vi "Max-SP-GetChannelRefs.vi"(8 "Error In":errorcluster, 9 "Enabled?":bool, 11 "Device Ref in":T1 format="%.0x") -> (0 "Error Out":errorcluster, 2 "Group Data Array":T2(array[cluster]) {"VS Refs" format="%.0x"}, 3 "Device Ref out":T1=18446744073709551615 format="%.0x")   [LabVIEW 2017, in "Waveform-Processing-Custom-Device Shared.lvlib" / "Max_SP.lvlib"]
uses:
  Max_SP.lvlib
  <vilib>/NI Veristand/Custom Device API/Custom Device Item Ref.ctl
  Constants.vi
  <vilib>/NI Veristand/Custom Device API/Get Item Property (Dependent Node Pointer).vi
  <vilib>/NI Veristand/Custom Device API/Custom Device API.lvlib
  System Explorer/Waveform-Processing-Custom-Device System Explorer.lvlib
  Waveform-Processing-Custom-Device Shared.lvlib
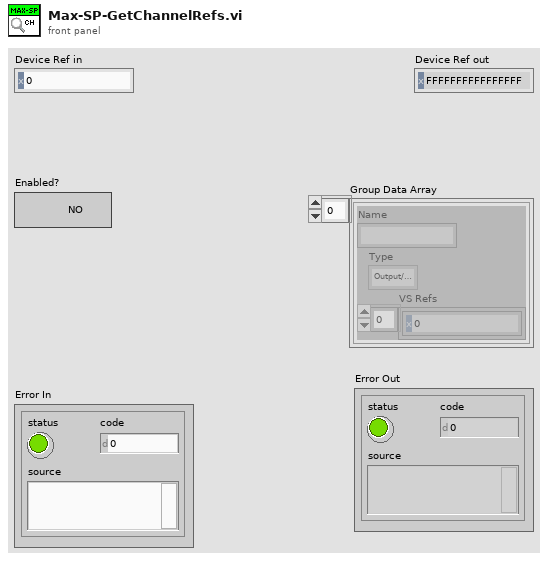
[diagram p1: front panel]
types:
  T1 = typedef "Custom Device API.lvlib/Custom Device Item Ref.ctl" = u64
  T2 = cluster{"Name":string, "Type":enum16{"Output/Write", "Input/Read", "Input/ReadWrite"}, "VS Refs":T1[]}[]
  T3 = enum16{"Output/Write", "Input/Read", "Input/ReadWrite"}
  T4 = cluster{"Name":string, "Type":enum16{"Output/Write", "Input/Read", "Input/ReadWrite"}, "VS Refs":T1[]}
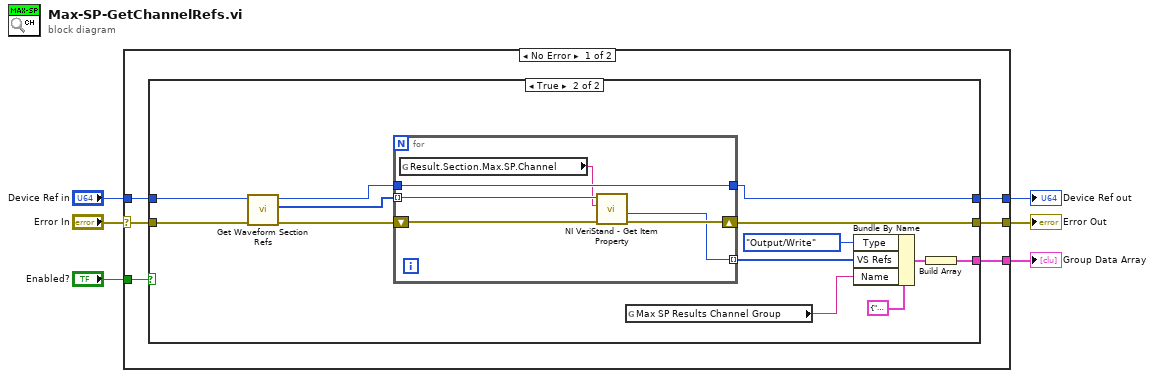
[diagram p0: block diagram]
diagram:
  n1 = case shown="No Error" "Error In" {
    selector: "Error In" -> [w12 w35]
    tunnel: [w10 w35] -> w2
    tunnel: "Device Ref in" -> [w11 w34]
    tunnel: "Enabled?" -> [w9 _]
    tunnel: [w8 w34] -> w1
    tunnel: [w7 _] -> w3
    frame No Error {
      n2 = case shown="True" w9 {
        tunnel: w12 -> [w14 w27]
        tunnel: w11 -> [w13 w26]
        tunnel: [w14 w22] -> w10
        tunnel: [w13 w21] -> w8
        tunnel: [_ w15] -> w7
        frame False {
        }
        frame True {
          n3 = call "Get Waveform Section Refs.vi"("Error in"=w27, "Device Ref in"=w26) -> ("Error out"=w25:errorcluster, "Result Section Refs"=w24:T1[], "Device Ref out"=w23:T1)  [unwired: 7 in]
          n4 = for {
            tunnel: w24 -> [w32] mode=indexing
            tunnel: w23 -> [w29]
            shift-right: [w31] -> w22
            shift-left: w25 -> [w33]
            tunnel: [w30] -> w20 mode=indexing
            tunnel: [w29] -> w21
            n5 = global read "Constants.vi" "Result.Section.Max.SP.Channel"() -> (w28:string)
            n6 = call-poly <vilib>:"NI VeriStand - Get Item Property.vi"("error in (no error)"=w33, "Property Name"=w28, "Item Ref in"=w32) -> ("error out"=w31:errorcluster, "Dependent Node Ref"=w30:T1)  [unwired: 5 in, 2 out]
          }
          n7 = global read "Constants.vi" "Max SP Results Channel Group"() -> (w17:string)
          n8 = Bundle By Name(cluster=T4 {"Name"="", "Type"=enum."Output/Write", "VS Refs"=[]} ("Group"), "Type"=T3."Output/Write", "VS Refs"=w20, "Name"=w17) -> (w16:T4)
          n9 = Build Array(w16) -> (w15:T2)
        }
      }
    }
    frame Error {
    }
  }
  "Device Ref out" <- w1
  "Group Data Array" <- w3
  "Error Out" <- w2
